vi "RunTimeObjectsSectionUI.vi"() -> ()   [LabVIEW 2015, in "RunTimeObjectsSection.lvclass"]
uses:
  RunTimeObjectsSection.lvclass
  <vilib>/NI/Configuration Framework/Node/NodeRef.ctl
  <vilib>/NI/Configuration Framework/Node/NISE_CEF_Node.lvclass
  <vilib>/NI/AMC/Message Queue.ctl
  <vilib>/NI/AMC/Message.ctl
  <vilib>/NI/Tools/Keyed Array/KeyedArray.ctl
  <vilib>/NI/Configuration Framework/Node/UserEventRef.ctl
  <vilib>/NI/Configuration Framework/Controls/EventCluster.ctl
  <vilib>/Utility/sysdir.llb/System Directory Type.ctl
  Custom Device Type Defs/RunTimeObjectTypes.ctl
  RunTimeObjectsSection.lvclass/RunTimeObjectsSection.ctl
  Read RunTimeObjectType.vi
  subVI/Config Global.vi
  <vilib>/NI/AMC/AMC.lvlib
  Configuration Tool.lvlib
  <vilib>/NI/Tools/Keyed Array/Tools_KeyedArray.lvlib
  <vilib>/NI/Configuration Framework/NISE_CEF_TreeControl.lvlib
panel:
  in  "WebBrowser":refnum<k7>(container)
  in  "user event":T1
  in  "main queue":T2
  in  "node ref":T3
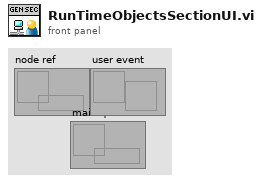
[diagram p1: front panel]
types:
  T1 = typedef "NISE_CEF_Node.lvclass/UserEventRef.ctl" = refnum<user-event>
  T2 = typedef "AMC.lvlib/Message Queue.ctl" = refnum<queue>
  T3 = typedef "NISE_CEF_Node.lvclass/NodeRef.ctl" = refnum<data-value>
  T4 = typedef "RunTimeObjectTypes.ctl" = enum16{"ActionVIs", "ButtonList", "RunTimeMenu"}
  T5 = typedef "System Directory Type.ctl" = i32
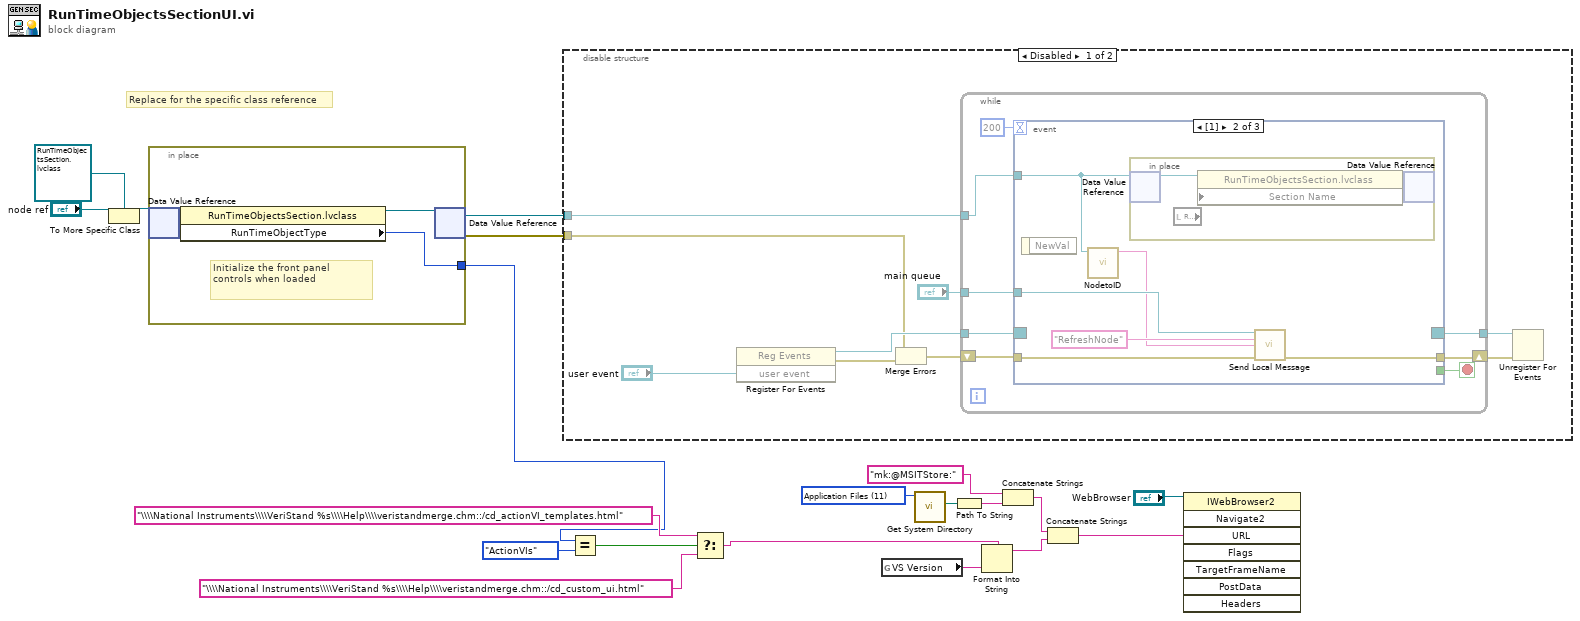
[diagram p0: block diagram]
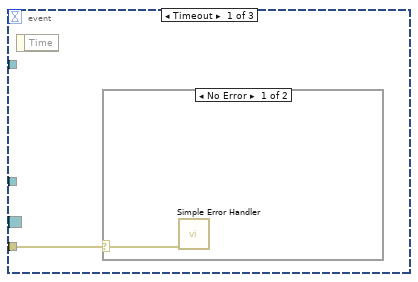
[diagram p2: hidden frame]
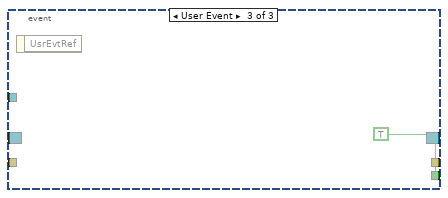
[diagram p4: hidden frame]
diagram:
  w20 = T5 11 items=["User Home"=0, "User Desktop"=1, "User Documents"=2, "User Application Data"=3, "User Preferences"=4, "User Temporary"=5, "Public Documents"=6, "Public Application Data"=7, "Public Preferences"=8, "Public Cache"=13, "System Core Libraries"=9, "System Installed Libraries"=10, "Application Files"=11, "Boot Volume Root"=12] ("system directory type")
  # "Replace for the specific class reference"
  n1 = To More Specific Class(target class=refnum<data-value> refnum ("data value reference"), reference="node ref") -> (specific class reference=w10:refnum<data-value>)  [unwired: 1 in, 1 out]
  n2 = in-place {
    in-place-border: [w21] -> w1
    # "Initialize the front panel controls when loaded"
    n3 = in-place-dvr #1(w10) -> (w23:refnum<class "RunTimeObjectsSection.lvclass">)  [unwired: 1 out]
    n4 = property class="RunTimeObjectsSection.lvclass"(reference=w23) -> (reference out=w22:refnum<class "RunTimeObjectsSection.lvclass">, "RunTimeObjectType"=w21:T4)  [unwired: 1 in, 1 out]
    n5 = in-place-dvr #1(w22) -> (w12:refnum<data-value>, w8:errorcluster)
  }
  n6 = disable-structure shown="Disabled" {
    disable-tunnel: w12 -> [w32 _]
    disable-tunnel: w8 -> [w25 _]
    frame Disabled {
      n7 = register-events("user event") -> (reference out=w29:refnum<event-registration>, error out=w26:errorcluster)  [unwired: 2 in]
      n8 = Merge Errors(w25, w26) -> (w24:errorcluster)
      n9 = while {
        tunnel: w32 -> [w40]
        tunnel: "main queue" -> [w39]
        tunnel: w29 -> [w37]
        tunnel: [w36] -> w28
        shift-right: [w34] -> w27
        shift-left: w24 -> [w33]
        stop <- w35 stop-if-true
        n10 = event shown="[1]" {
          selector: w37 -> [_ _ _]
          dyn-events: [_ _ _] -> w36
          timeout: 200 -> [_ _ _]
          tunnel: w40 -> [_ w46 _]
          tunnel: w39 -> [_ w47 _]
          tunnel: [_ _ TRUE] -> w35
          tunnel: [_ w44 _] -> w34
          tunnel: w33 -> [w41 w43 _]
          event Timeout {
            n11 = event-data() -> ()  [unwired: 1 in, 1 out]
            n12 = case shown="No Error" w41 {
              selector: w41 -> [w42 _]
              frame No Error {
                n13 = call <vilib>:"Simple Error Handler.vi"("error in (no error)"=w42) -> ()  [unwired: 4 in, 5 out]
              }
              frame Error {
              }
            }
          }
          event #1 (no event record) {
            n14 = event-data() -> ()  [unwired: 1 in, 1 out]
            n15 = call <vilib>:"NodetoID.vi"("node ref"=w46) -> ("ID"=w45:string)  [unwired: 9 in, 1 out]
            n16 = in-place {
              n17 = in-place-dvr #2(w46) -> (w50:refnum<class "RunTimeObjectsSection.lvclass">)  [unwired: 1 out]
              n18 = local read item#-1() -> ()  [unwired: 1 out]
              n19 = property class="RunTimeObjectsSection.lvclass" props=["Section Name"](reference=w50) -> (reference out=w49:refnum<class "RunTimeObjectsSection.lvclass">)  [unwired: 2 in, 1 out]
              n20 = in-place-dvr #2(w49) -> ()  [unwired: 2 out]
            }
            n21 = call <vilib>:"Send Local Message.vi"("message queue in"=w47, "message name"="RefreshNode" ("Message Name"), "message value"=w45, "error in"=w43) -> ("error out"=w44:errorcluster)  [unwired: 9 in, 2 out]
          }
          event User Event {
            n22 = event-data() -> ()  [unwired: 1 in, 1 out]
          }
        }
      }
      n23 = Unregister For Events(event registration refnum=w28, error in=w27) -> ()  [unwired: 1 out]
    }
    frame Enabled {
    }
  }
  n24 = Equal?(x=w1, y=RunTimeObjectTypes."ActionVIs") -> (x = y?=w5:bool)
  n25 = Select(t="\\\\National Instruments\\\\VeriStand %s\\\\Help\\\\veristandmerge.chm::/cd_actionVI_templates.html", s=w5, f="\\\\National Instruments\\\\VeriStand %s\\\\Help\\\\veristandmerge.chm::/cd_custom_ui.html") -> (s? t:f=w3:string)
  n26 = global read "Config Global.vi" "VS Version"() -> (w13:string)
  n27 = call <vilib>:"Get System Directory.vi"("system directory type"=w20) -> ("system directory"=w19:path)  [unwired: 10 in]
  n28 = Path To String(path=w19) -> (string=w18:string)
  n29 = Format Into String(format string=w3, w13) -> (resulting string=w15:string)  [unwired: 2 in, 1 out]
  n30 = Concatenate Strings("mk:@MSITStore:" ("concatenated string"), w18) -> (w16:string)
  n31 = Concatenate Strings(w16, w15) -> (w2:string)
  n32 = invoke class="IWebBrowser2" method="Navigate2"(reference="WebBrowser", "URL"=w2) -> ()  [unwired: 6 in, 8 out]
